vi "Scale injector.vi"() -> (3 "Rare Field":dbl)   [LabVIEW 2016]
uses:
  Injector global.vi
panel:
  in  "stop":bool
  in  "Stable Injected Mass":dbl=1.0
  in  "Rare Injected Mass":dbl=1.0
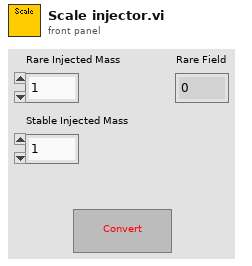
[diagram p1: front panel]
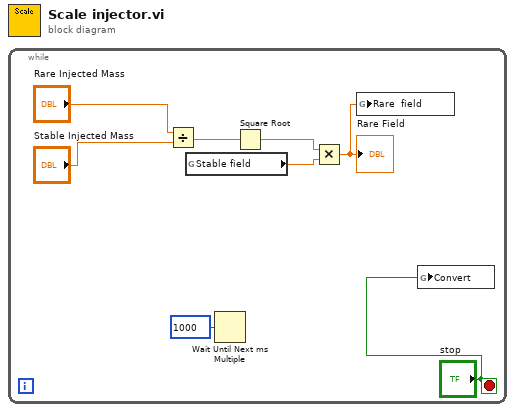
[diagram p0: block diagram]
diagram:
  n1 = while {
    stop <- "stop" stop-if-true
    n2 = Divide(x="Rare Injected Mass", y="Stable Injected Mass") -> (x/y=w6:dbl)
    n3 = global read "Injector global.vi" "Stable field"() -> (w5:dbl)
    n4 = Wait Until Next ms Multiple(millisecond multiple=u32 1000) -> ()  [unwired: 1 out]
    n5 = Square Root(x=w6) -> (sqrt(x)=w4:dbl)
    n6 = Multiply(x=w4, y=w5) -> (x*y=w3:dbl)
    "Rare Field" <- w3
    n7 = global write "Injector global.vi" "Rare  field"(w3) -> ()
    n8 = global write "Injector global.vi" "Convert"("stop") -> ()
  }
